vi "Get 335 Main Temp(SubVI).vi"(11 "队列输入":refnum<queue>) -> (0 "error out":errorcluster, 8 "Main Temp":dbl)   [LabVIEW 2019, in "SubVI.lvlib"]
uses:
  SubVI.lvlib
  config.ctl
  Instrument.ctl
  lib/QDInstrument.dll
  <vilib>/NI/Modbus Library/API/Master/Modbus Master.lvclass
  lib/Lake Shore 335/Lake Shore 335.lvlib
panel:
  # "(真是通道1，假是通道2)"
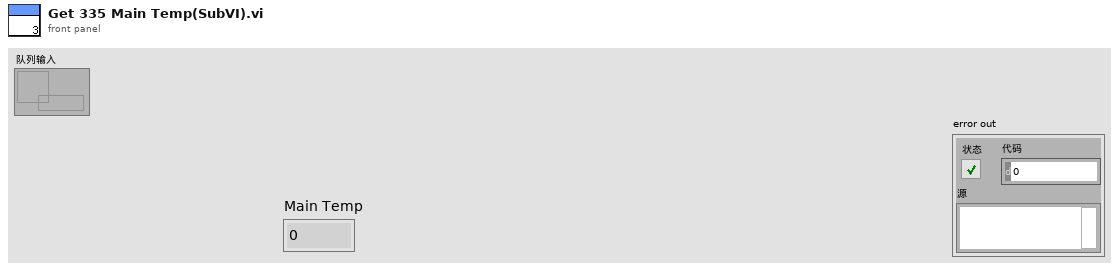
[diagram p1: front panel]
types:
  T1 = typedef "config.ctl" = cluster{"initialize":string, "6221":cluster{"6221 Resource":refnum<visa-resource-name>, "Delta status":bool}, "7001":cluster{"Ch":bool}, "SR830+6221":cluster{"source":u16, "阻抗":dbl, "量程入 4":i32, "量程入 3":i32, "量程入 2":i32, "量程入 1":i32, "电流":dbl, "SR830 2":bool, "SR830 3":bool, "SR830 4":bool, "SR830 1":bool, "VISA 1":refnum<visa-resource-name>, "VISA 2":refnum<visa-resource-name>, "VISA 3":refnum<visa-resource-name>, "VISA 4":refnum<visa-resource-name>, "量程":enum16{"量程每次测量会判定", "量程不变为设定值"}}, "2400":cluster{"2400":bool, "VISA":refnum<visa-resource-name>}, "ch":cluster{"ch str":string, "ch1":bool, "ch2":bool, "布尔":bool}, "error":bool, "数据文件路径":path, "log":cluster{"log路径":path, "log interval":dbl}, "Instrument":T2}
  T2 = typedef "Instrument.ctl" = cluster{"335 Resource":refnum<visa-resource-name>, "Input (0:A)":u16, "Instrument Type":i32, "quantum design":refnum<k24>, "Heater Output (1:1)":u16, "335state":refnum<vi>, "semaphore":T3, "TCP master instance":refnum<class "Modbus Master.lvclass">}
  T3 = typedef "Semaphore RefNum" = refnum<k1>
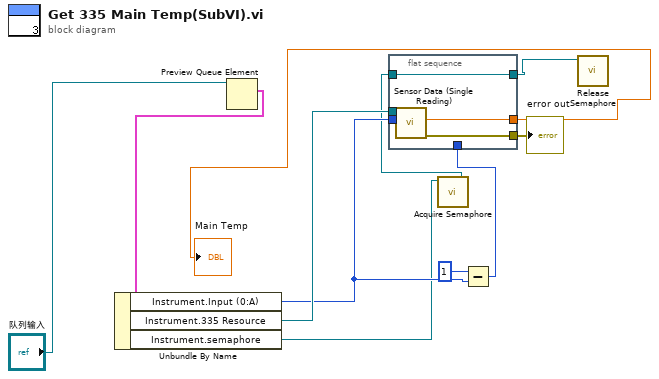
[diagram p0: block diagram]
diagram:
  n1 = Preview Queue Element(queue="队列输入") -> (element=w10:T1)  [unwired: 2 in, 3 out]
  n2 = Unbundle By Name(w10) -> ("Instrument.Input (0:A)"=w8:u16, "Instrument.335 Resource"=w9:refnum<visa-resource-name>, "Instrument.semaphore"=w7:T3)
  n3 = flat-sequence {
    tunnel: w9 -> [w16]
    tunnel: w8 -> [w15]
    tunnel: w5 -> [_]
    tunnel: [w14] -> w2
    tunnel: w4 -> [w13]
    tunnel: [w13] -> w3
    tunnel: [w12] -> w1
    frame #0 {
      n4 = call "Sensor Data (Single Reading).vi"("Input (0:A)"=w15, "VISA resource name"=w16) -> ("error out"=w12:errorcluster, "Sensor Data"=w14:dbl)  [unwired: 7 in, 1 out]
    }
  }
  n5 = call <vilib>:"Acquire Semaphore.vi"("semaphore"=w7) -> ("semaphore out"=w4:T3)  [unwired: 4 in, 2 out]
  n6 = Subtract(x=u16 1, y=w8) -> (x-y=w5:u16)
  n7 = call <vilib>:"Release Semaphore.vi"("semaphore"=w3) -> ()  [unwired: 5 in, 2 out]
  "Main Temp" <- w2
  "error out" <- w1
